vi "Read EnableOutput.ACT.vi"(8 "error in":errorcluster, 11 "Cycler in":refnum<class "Cycler.lvclass">) -> (0 "error out":errorcluster, 2 "EnableOutput.ACT":bool, 3 "Cycler out":refnum<class "Cycler.lvclass">)   [LabVIEW 2023, in "Cycler.lvclass"]
uses:
  Cycler.lvclass
  Cycler.lvclass/Cycler.ctl
  <vilib>/ADAS Replay HIL/Channels/Tag Wrapper/Tag Wrapper.lvlib
  <vilib>/ADAS Replay HIL/Channels/Tag Wrapper/Polymorphic/Read Channel (Boolean).vi
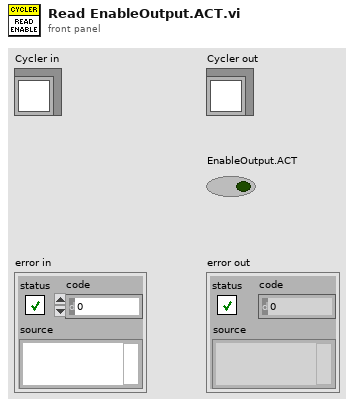
[diagram p1: front panel]
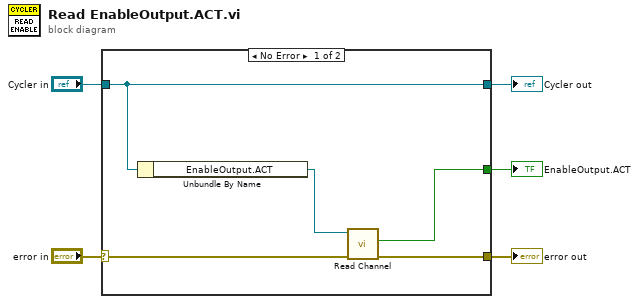
[diagram p0: block diagram]
diagram:
  n1 = case shown="No Error" "error in" {
    selector: "error in" -> [w9 w11]
    tunnel: [w8 w11] -> w4
    tunnel: [w10 w12] -> w2
    tunnel: "Cycler in" -> [w10 w12]
    tunnel: [w6 _] -> w1
    frame No Error {
      n2 = Unbundle By Name(w10) -> ("EnableOutput.ACT"=w7:refnum<k21>)
      n3 = call-poly <vilib>:"Read Channel.vi"("error in"=w9, "ADAS HIL Channel in"=w7) -> ("error out"=w8:errorcluster, "Value out"=w6:bool)  [unwired: 6 in, 2 out]
    }
    frame Error {
    }
  }
  "error out" <- w4
  "Cycler out" <- w2
  "EnableOutput.ACT" <- w1
